vi "Com_SECS Equipment _Control Message(Linktest).vi"(8 "error in":errorcluster, 10 "Timeout":i32=1000, 11 "Buffer Data In":T1) -> (0 "error out":errorcluster, 3 "Buffer Data Out":T1)   [LabVIEW 2016]
uses:
  Data Def/Com_SECS Equipment _Buffer Data.ctl
  Data Def/Com_SECS Equipment _Connection Setting.ctl
  Data Def/Com_SECS Equipment _Timeout Setting.ctl
  Data Def/Com_SECS Equipment _SECS Packet.ctl
  Data Def/Com_SECS Equipment _Message Type.ctl
  Data Def/Com_SECS Equipment _Protocol Type.ctl
  Data Def/Com_SECS Equipment _Stream Type.ctl
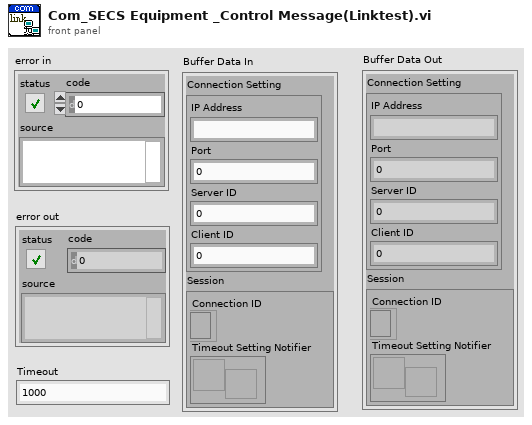
[diagram p1: front panel]
types:
  T1 = typedef "Com_SECS Equipment _Buffer Data.ctl" = cluster{"Connection Setting":T2, "Session":cluster{"Connection ID":refnum<k5>, "Timeout Setting Notifier":refnum<notifier>}}
  T2 = typedef "Com_SECS Equipment _Connection Setting.ctl" = cluster{"IP Address":string, "Port":u16, "Server ID":u16, "Client ID":u16}
  T3 = typedef "Com_SECS Equipment _Stream Type.ctl" = enum16{"Data Message", "Select.req", "Select.rsp", "Deselect.req", "Deselect.rsp", "Linktest.req", "Linktest.rsp", "Reject.req", "Separate.req", "Reserve"}
  T4 = typedef "Com_SECS Equipment _SECS Packet.ctl" = cluster{"Need Response?":bool, "Device ID":u16, "Stream":u8, "Function":u8, "Message Type":T5, "Protocol Type":T6, "Stream Type":T3, "System Btyes":u8[], "Message Data":u8[]}
  T5 = typedef "Com_SECS Equipment _Message Type.ctl" = enum16{"Control Message", "Data Message"}
  T6 = typedef "Com_SECS Equipment _Protocol Type.ctl" = enum16{"SECS-II Encoding", "Reserved"}
  T7 = typedef "Com_SECS Equipment _Timeout Setting.ctl" = cluster{"T3(Reply Timeout)":dbl, "T5(Separation Timeout)":dbl, "T6(Control Timeout)":dbl, "T7(Not Selected Timeout)":dbl, "T8(Inter-Character Timeout)":dbl}
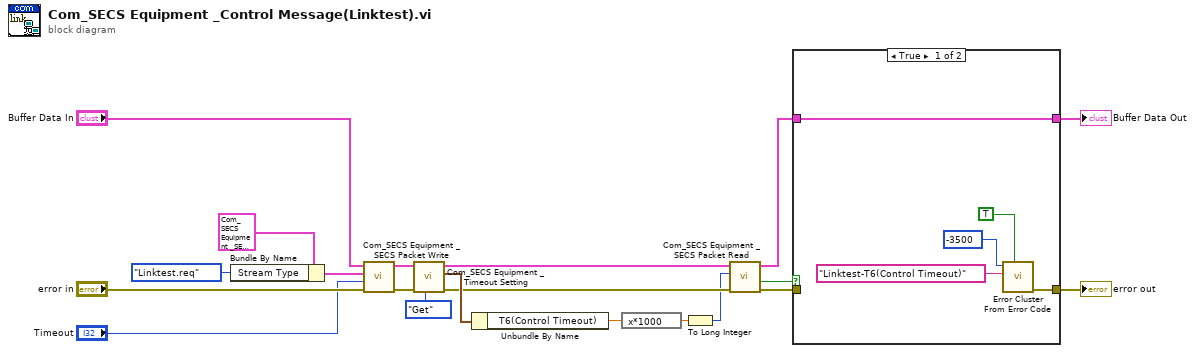
[diagram p0: block diagram]
diagram:
  n1 = Bundle By Name(cluster=T4 {"Need Response?"=FALSE, "Device ID"=0, "Stream"=0, "Function"=0, "Message Type"=enum."Control Message", "Protocol Type"=enum."SECS-II Encoding", "Stream Type"=enum."Linktest.req", "System Btyes"=[], "Message Data"=[]} ("SECS Packet"), "Stream Type"=Com_SECS_Equipment__Stream_Type."Linktest.req") -> (w7:T4)
  n2 = call "Com_SECS Equipment _SECS Packet Write.vi"("error in"="error in", "Timeout"="Timeout", "SECS Packet"=w7, "Buffer Data In"="Buffer Data In") -> ("error out"=w11:errorcluster, "Buffer Data Out"=w12:T1)  [unwired: 6 in]
  n3 = call "Com_SECS Equipment _Timeout Setting.vi"("Method"=enum16{"Get", "Put"}."Get", "error in"=w11, "Buffer Data In"=w12) -> ("error out"=w6:errorcluster, "Timeout Setting Out"=w19:T7, "Buffer Data Out"=w4:T1)  [unwired: 6 in]
  n4 = Unbundle By Name(w19) -> ("T6(Control Timeout)"=w18:dbl)
  n5 = expression code="x*1000"(w18) -> (w17:dbl)
  n6 = To Long Integer(number=w17) -> (32bit integer=w5:i32)
  n7 = call "Com_SECS Equipment _SECS Packet Read.vi"("error in"=w6, "Timeout(100)"=w5, "Buffer Data In"=w4) -> ("error out"=w3:errorcluster, "Timeout?"=w2:bool, "Buffer Data Out"=w1:T1)  [unwired: 5 in, 1 out]
  n8 = case shown="True" w2 {
    tunnel: w1 -> [w25 w27]
    tunnel: [w25 w27] -> w16
    tunnel: [w21 w26] -> w15
    tunnel: w3 -> [_ w26]
    frame True {
      n9 = call <vilib>:"Error Cluster From Error Code.vi"("show call chain? (False)"=TRUE, "error message (\"\")"="Linktest-T6(Control Timeout)" ("error message (\"\")"), "error code (0)"=-3500) -> ("error out"=w21:errorcluster)  [unwired: 6 in]
    }
    frame False {
    }
  }
  "error out" <- w15
  "Buffer Data Out" <- w16
